vi "Check Home Init Status.vi"(5 "Status Byte":u16) -> (6 "Home Init?":bool)   [LabVIEW 2015, in "Tool Module.lvlib"]
uses:
  Tool Module.lvlib
  _Status Bits Typedef.ctl
  Tool Config/Tool Cfg.lvlib
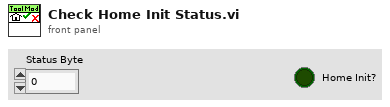
[diagram p1: front panel]
types:
  T1 = typedef "Tool Module.lvlib/_Status Bits Typedef.ctl" = u16
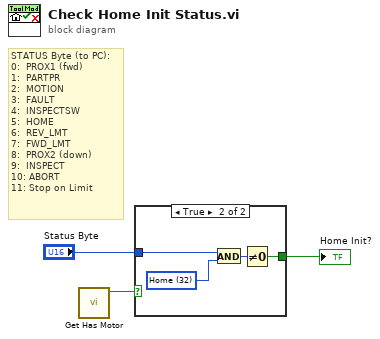
[diagram p0: block diagram]
diagram:
  # "STATUS Byte (to PC):\n0:  PROX1 (fwd)\n1:  PARTPR\n2:  MOTION\n3:  FAULT\n4:  INSPECTSW\n5:  HOME\n6:  REV_LMT\n7:  FWD_LMT\n8:  PROX2 (down)\n9:  INSPECT\n10: ABORT\n11: Stop on Limit"
  n1 = call "Get Has Motor.vi"() -> ("Has Motor"=w1:bool)  [unwired: 11 in]
  n2 = case shown="True" w1 {
    tunnel: [_ w6] -> w3
    tunnel: "Status Byte" -> [_ w5]
    frame False {
    }
    frame True {
      w4 = T1 32 items=["PROX1"=1, "PartPresent"=2, "Motion"=4, "Fault"=8, "Switch"=16, "Home"=32, "RLS"=64, "FLS"=128, "PROX2"=256, "INSPECT"=512, "Abort"=1024, "Stop on Limit"=2048] ("_Status bit values typedef")
      n3 = And(x=w5, y=w4) -> (x .and. y?=w7:T1)
      n4 = Not Equal To 0?(x=w7) -> (x != 0?=w6:bool)
    }
  }
  "Home Init?" <- w3
